vi "GEA3 Write Gains.vi"(0 "Kp Gain Value":i32, 1 "Convert to HEX?":bool, 5 "Kp Qbits Value":i32, 7 "Ki Gain Value":i32, 9 "Ki Qbits Value":i32, 11 "Gain Data Input":string) -> (4 "Gain Data Output":string, 6 "Kp Gain Out":i32, 8 "Kp Qbits Out":i32, 10 "Ki Gain Out":i32, 15 "Ki Qbits Out":i32)   [LabVIEW 2020]
uses:
  library/GEA2_Toolkit.lvlib
panel:
  # "Convert to HEX"
  # "Convert to Values"
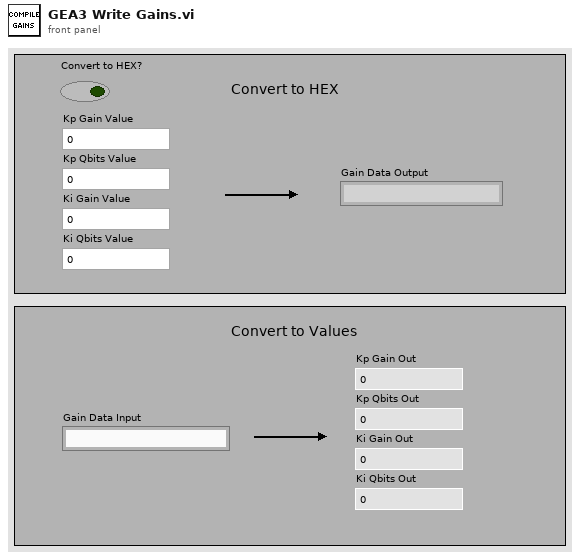
[diagram p1: front panel]
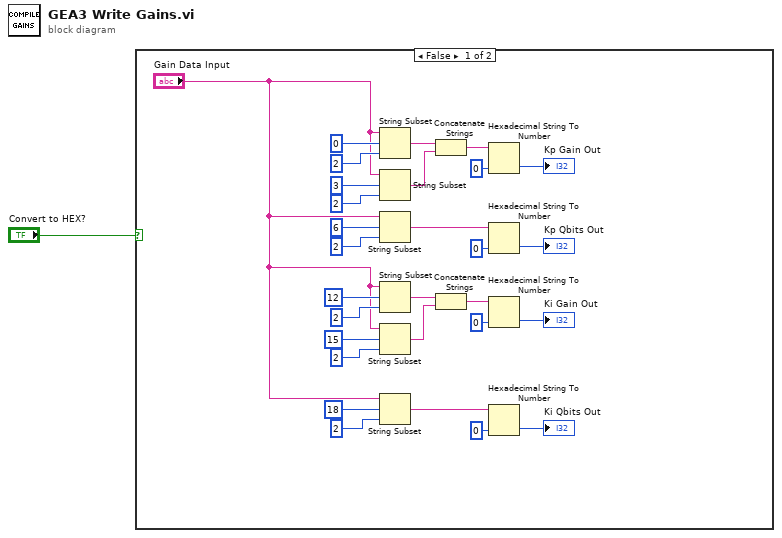
[diagram p0: block diagram]
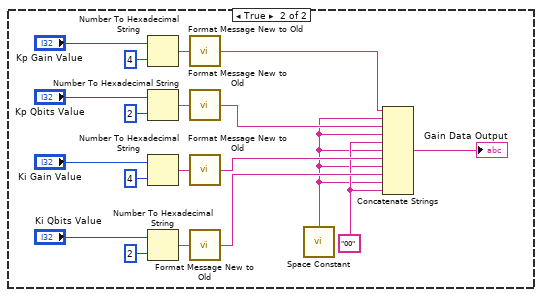
[diagram p2: hidden frame]
diagram:
  n1 = case shown="False" "Convert to HEX?" {
    frame False {
      n2 = String Subset(string="Gain Data Input", offset (0)=0, length (rest)=2 ("length (rest)")) -> (substring=w27:string)
      n3 = String Subset(string="Gain Data Input", offset (0)=3, length (rest)=2 ("length (rest)")) -> (substring=w26:string)
      n4 = String Subset(string="Gain Data Input", offset (0)=6, length (rest)=2 ("length (rest)")) -> (substring=w18:string)
      n5 = String Subset(string="Gain Data Input", offset (0)=12, length (rest)=2 ("length (rest)")) -> (substring=w12:string)
      n6 = String Subset(string="Gain Data Input", offset (0)=15, length (rest)=2 ("length (rest)")) -> (substring=w13:string)
      n7 = String Subset(string="Gain Data Input", offset (0)=18, length (rest)=2 ("length (rest)")) -> (substring=w7:string)
      n8 = Concatenate Strings(w27, w26) -> (w24:string)
      n9 = Concatenate Strings(w12, w13) -> (w15:string)
      n10 = Hexadecimal String To Number(string=w24, default (0uL)=0 ("default (0 U32)")) -> (number=→"Kp Gain Out":i32)  [unwired: 1 in, 1 out]
      n11 = Hexadecimal String To Number(string=w18, default (0uL)=0 ("default (0 U32)")) -> (number=→"Kp Qbits Out":i32)  [unwired: 1 in, 1 out]
      n12 = Hexadecimal String To Number(string=w15, default (0uL)=0 ("default (0 U32)")) -> (number=→"Ki Gain Out":i32)  [unwired: 1 in, 1 out]
      n13 = Hexadecimal String To Number(string=w7, default (0uL)=0 ("default (0 U32)")) -> (number=→"Ki Qbits Out":i32)  [unwired: 1 in, 1 out]
    }
    frame True {
      w32 = "00"
      n14 = Number To Hexadecimal String(1:i16 4 ("width (-)"), 2:"Kp Gain Value") -> (0:w35:string)
      n15 = Number To Hexadecimal String(1:i16 2 ("width (-)"), 2:"Kp Qbits Value") -> (0:w39:string)
      n16 = Number To Hexadecimal String(1:i16 4 ("width (-)"), 2:"Ki Gain Value") -> (0:w45:string)
      n17 = Number To Hexadecimal String(1:i16 2 ("width (-)"), 2:"Ki Qbits Value") -> (0:w42:string)
      n18 = call "Format Message New to Old.vi"("Raw Message In"=w35) -> ("Conv Message Out"=w46:string)  [unwired: 14 in]
      n19 = call "Format Message New to Old.vi"("Raw Message In"=w39) -> ("Conv Message Out"=w47:string)  [unwired: 14 in]
      n20 = call "Format Message New to Old.vi"("Raw Message In"=w45) -> ("Conv Message Out"=w48:string)  [unwired: 14 in]
      n21 = call "Format Message New to Old.vi"("Raw Message In"=w42) -> ("Conv Message Out"=w33:string)  [unwired: 14 in]
      n22 = call <vilib>:"Space Constant.vi"() -> ("String"=w31:string)
      n23 = Concatenate Strings(w46, w31, w47, w31, w32, w31, w48, w31, w33, w31, w32) -> (→"Gain Data Output":string)
    }
  }
